vi "Write data to Signal Ref.vi"(8 "error in (no error)":errorcluster, 10 "Waveform Graph":dynamicdata(graph), 11 "Data Saver in":refnum<class "Data Saver.lvclass">) -> (0 "error out":errorcluster, 3 "Data Saver out":refnum<class "Data Saver.lvclass">)   [LabVIEW 2016, in "Data Saving.lvlib" / "Data Saver.lvclass"]
uses:
  Data Saver.lvclass
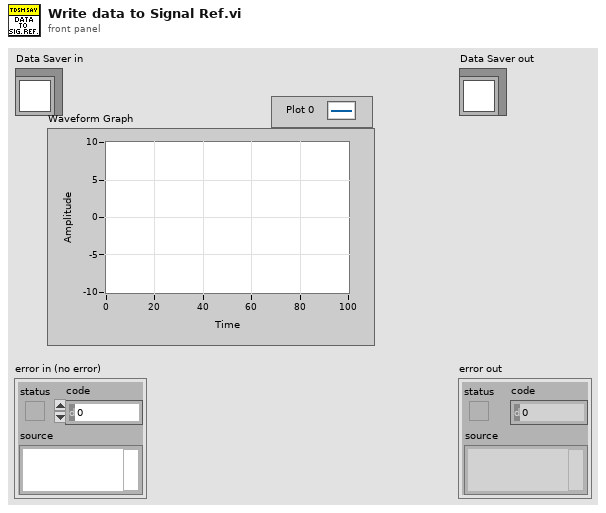
[diagram p1: front panel]
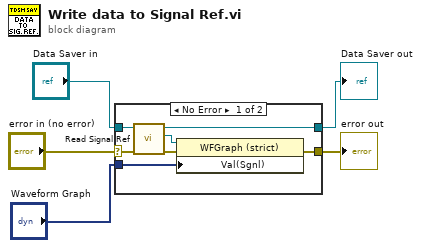
[diagram p0: block diagram]
diagram:
  n1 = case shown="No Error" "error in (no error)" {
    selector: "error in (no error)" -> [w10 w14]
    tunnel: [w6 w14] -> w4
    tunnel: [w11 w13] -> w2
    tunnel: "Data Saver in" -> [w12 w13]
    tunnel: "Waveform Graph" -> [w7 _]
    frame No Error {
      n2 = call-dynamic "Read Signal Ref.vi"("error in (no error)"=w10, "Abstract Saver in"=w12) -> ("error out"=w8:errorcluster, "Signal Ref"=w9:refnum<vi>, "Abstract Saver out"=w11:refnum<class "Data Saver.lvclass">)  [unwired: 7 in]
      n3 = property class="WFGraph (strict)"(reference=w9, error in=w8, "Val(Sgnl)"=w7) -> (error out=w6:errorcluster)  [unwired: 1 out]
    }
    frame Error {
    }
  }
  "error out" <- w4
  "Data Saver out" <- w2
